vi "EventHandleInstrumentStatusChanged.vi"(4 "User Parameter":variant, 5 "Event Data":cluster{"sender":refnum<k24>, "e":refnum<k24>}, 6 "Control Ref":refnum<k24>, 7 "Event Common Data":T1) -> ()   [LabVIEW 2014]
uses:
  C:/Program Files (x86)/Molecular Devices/SoftMax Pro 6.5.1 Automation SDK/SoftMaxPro.AutomationClient.dll
  Program Files (x86)/Molecular Devices/SoftMax Pro 6.5.1 Automation SDK/SoftMaxPro.AutomationClient.dll
  EventHandleInstrumentStatusChangedData.ctl
  PlateReaderGlobal.vi
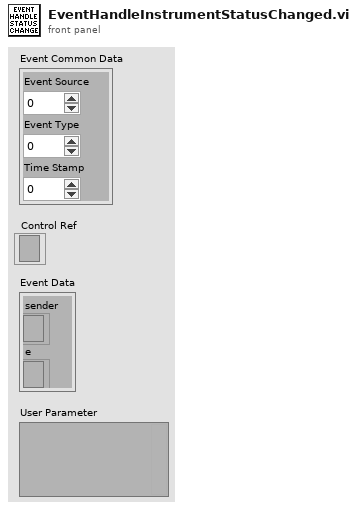
[diagram p1: front panel]
types:
  T1 = cluster{"Event Source":i32, "Event Type":u32, "Time Stamp":u32}
  T2 = typedef "EventHandleInstrumentStatusChangedData.ctl" = cluster{"Event Common Data":cluster{"Event Source":i32, "Event Type":u32, "Time Stamp":u32}, "Status":string}
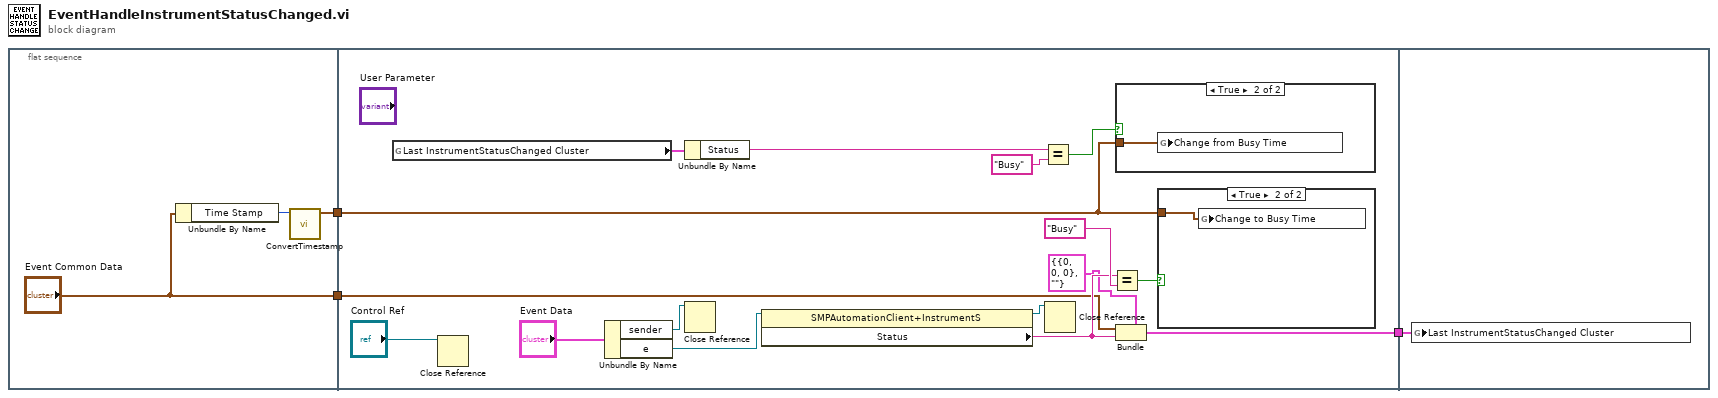
[diagram p0: block diagram]
diagram:
  n1 = flat-sequence {
    tunnel: ["Event Common Data"] -> w3
    tunnel: [w4] -> w1
    tunnel: w3 -> [w9]
    tunnel: [w8] -> w2
    tunnel: w1 -> [w7]
    tunnel: w2 -> [w25]
    frame #0 {
      n2 = Unbundle By Name("Event Common Data") -> ("Time Stamp"=w6:u32)
      n3 = call "ConvertTimestamp.vi"("Time Stamp"=w6) -> ("Timestamp"=w4:timestamp)  [unwired: 10 in]
    }
    frame #1 {
      n4 = global read "PlateReaderGlobal.vi" "Last InstrumentStatusChanged Cluster"() -> (w22:T2)
      n5 = Close Reference(reference="Control Ref") -> ()  [unwired: 1 in, 1 out]
      n6 = Unbundle By Name("Event Data") -> ("sender"=w13:refnum<k24>, "e"=w11:refnum<k24>)
      n7 = Unbundle By Name(w22) -> ("Status"=w20:string)
      n8 = Close Reference(reference=w13) -> ()  [unwired: 1 in, 1 out]
      n9 = property class="SMPAutomationClient+InstrumentS"(reference=w11) -> (reference out=w14:refnum<k24>, "Status"=w15:string)  [unwired: 1 in, 1 out]
      n10 = Equal?(x=w20, y="Busy") -> (x = y?=w19:bool)
      n11 = Close Reference(reference=w14) -> ()  [unwired: 1 in, 1 out]
      n12 = Equal?(x=w15, y="Busy") -> (x = y?=w17:bool)
      n13 = case shown="True" w19 {
        tunnel: w7 -> [_ w23]
        frame False {
        }
        frame True {
          n14 = global write "PlateReaderGlobal.vi" "Change from Busy Time"(w23) -> ()
        }
      }
      n15 = Bundle(cluster=T2 {"Event Common Data"={"Event Source"=0, "Event Type"=0, "Time Stamp"=0}, "Status"=""} ("Event Data Cluster"), "Event Common Data"=w9, "Status"=w15) -> (w8:T2)
      n16 = case shown="True" w17 {
        tunnel: w7 -> [_ w24]
        frame False {
        }
        frame True {
          n17 = global write "PlateReaderGlobal.vi" "Change to Busy Time"(w24) -> ()
        }
      }
    }
    frame #2 {
      n18 = global write "PlateReaderGlobal.vi" "Last InstrumentStatusChanged Cluster"(w25) -> ()
    }
  }
